vi "Read Channels and optional channel names.vi"(11 "Switching Time in":refnum<class "Switching Time.lvclass">) -> (2 "Channels and optional channel names":cluster{"Enabled":bool, "Channel name":string}[](array[cluster])=[{"Enabled"=TRUE, "Channel name"=""}, {"Enabled"=FALSE, "Channel name"=""}, {"Enabled"=FALSE, "Channel name"=""}, {"Enabled"=FALSE, "Channel name"=""}], 3 "Switching Time out":refnum<class "Switching Time.lvclass">)   [LabVIEW 2020, in "Switching Time.lvclass"]
uses:
  Switching Time.lvclass
  Switching Time.lvclass/Switching Time.ctl
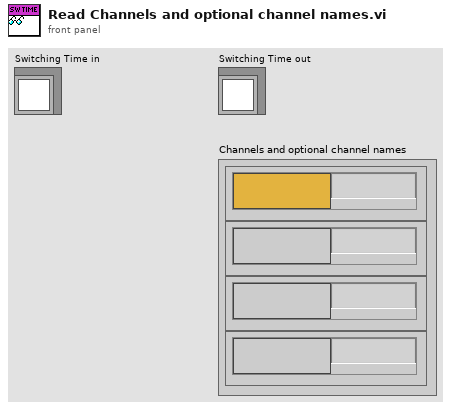
[diagram p1: front panel]
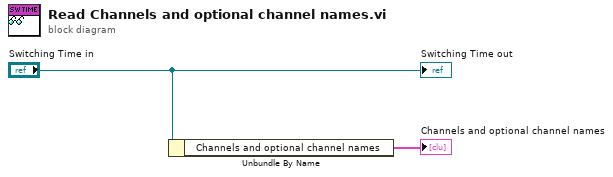
[diagram p0: block diagram]
diagram:
  n1 = Unbundle By Name("Switching Time in") -> ("Channels and optional channel names"=→"Channels and optional channel names":cluster{"Enabled":bool, "Channel name":string}[])
  "Switching Time out" <- "Switching Time in"
